vi "Resize Image for Question.vi"(8 "error in (no error)":errorcluster, 11 "Controller in":refnum<class "Controller.lvclass">) -> (0 "error out":errorcluster, 3 "Controller Out":refnum<class "Controller.lvclass">)   [LabVIEW 2024, in "Controller.lvlib" / "Controller.lvclass"]
uses:
  Controller.lvclass
  Controller.lvclass/Controller.ctl
  <vilib>/picture/picture.llb/Draw True-Color Pixmap.vi
  <vilib>/Dataflow_G/G-Image/Image Processing/Polymorphic VIs/Resize Image (Scale).vi
  <vilib>/Dataflow_G/G-Image/G-Image.lvlib
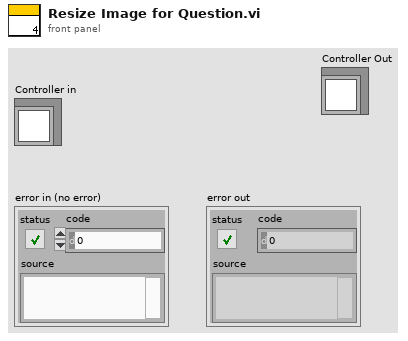
[diagram p1: front panel]
types:
  T1 = cluster{"horizontal":enum16{"left", "center", "right"}, "vertical":enum16{"top", "center", "bottom"}, "text":enum16{"left", "center", "right"}}
  T2 = enum16{"User-specified Font", "Application Font", "System Font", "Dialog Font"}
  T3 = cluster{"Font Name:":string, "Size":i16, "Strikeout?":bool, "Italic?":bool, "Underline?":bool, "Outline?":bool, "Shadow?":bool, "Bold?":bool}
  T4 = cluster{"left":i16, "top":i16, "right":i16, "bottom":i16}
  T5 = typedef "imagedata.ctl" = cluster{"image type":i32, "image depth":i32, "image":u8[], "mask":u8[], "colors":u32[], "Rectangle":cluster{"left":i16, "top":i16, "right":i16, "bottom":i16}}
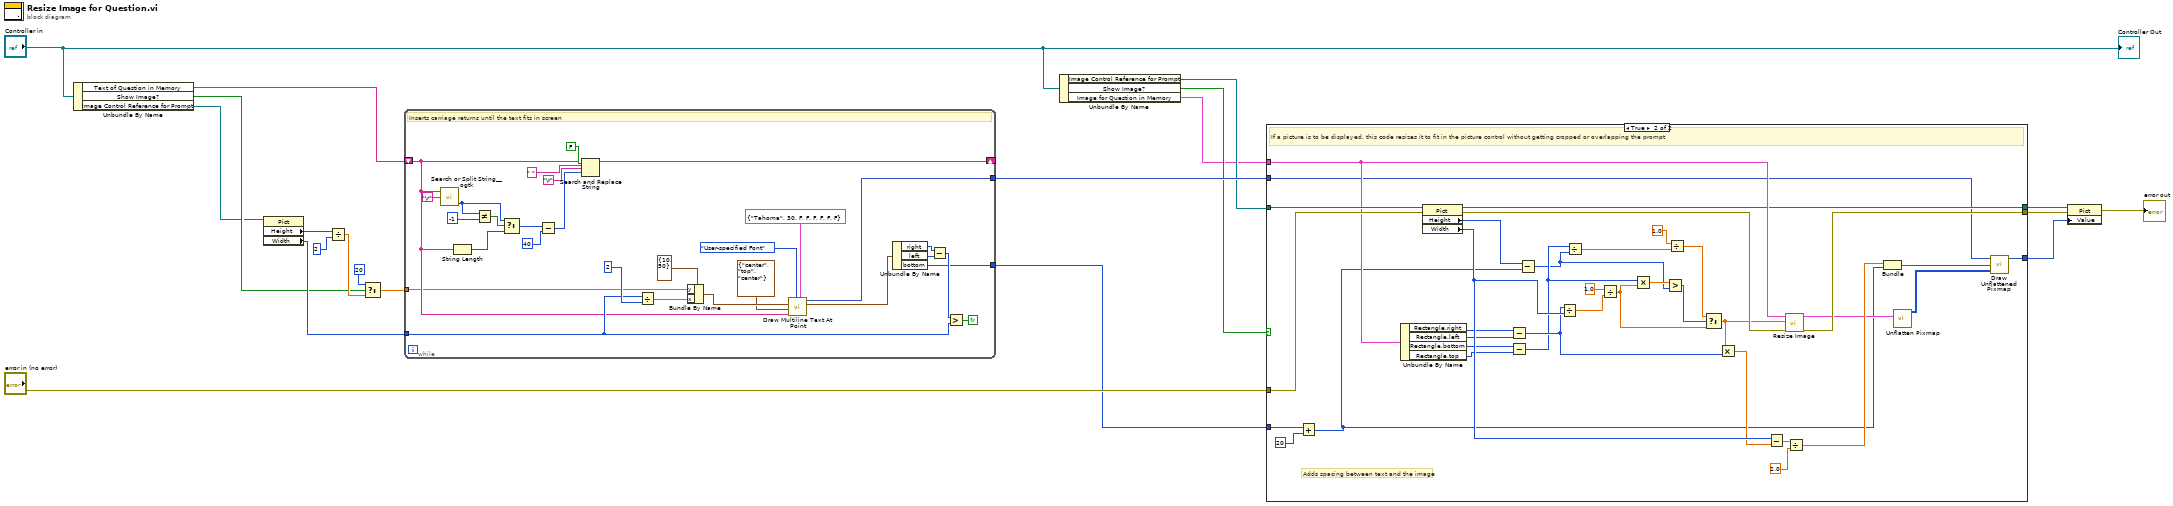
[diagram p0: block diagram]
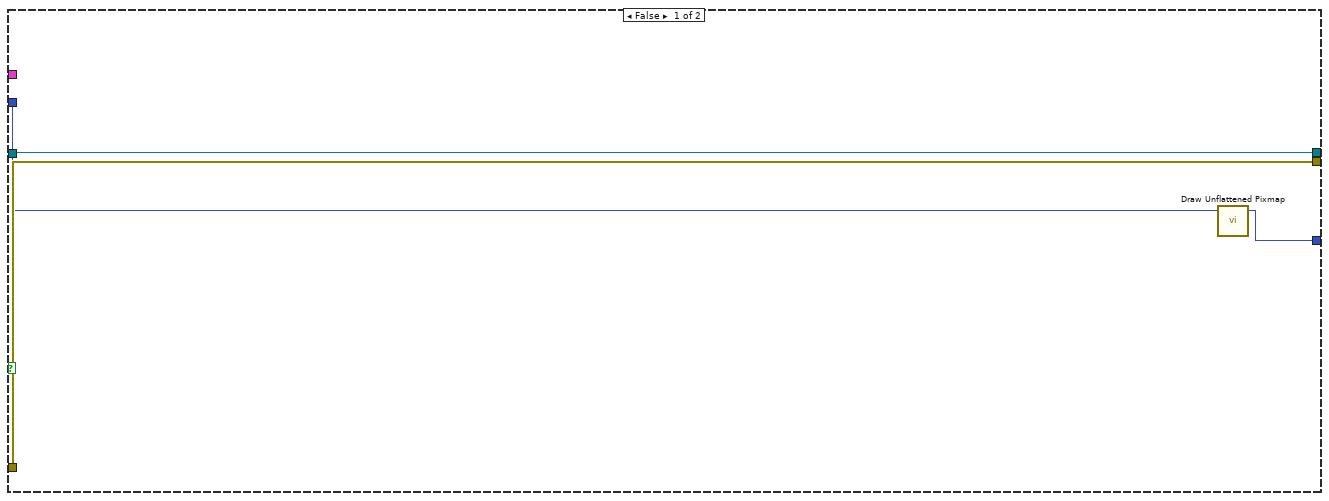
[diagram p2: hidden frame]
diagram:
  n1 = Unbundle By Name("Controller in") -> ("Text of Question in Memory"=w5:string, "Show Image?"=w4:bool, "Image Control Reference for Prompt"=w2:refnum<vi>)
  n2 = property class="Pict"(reference=w2) -> ("Height"=w8:u32, "Width"=w6:u32)  [unwired: 1 in, 2 out]
  n3 = Divide(x=w8, y=u32 2) -> (x/y=w7:dbl)
  n4 = Select(t=i16 20 ("x"), s=w4, f=w7) -> (s? t:f=w13:dbl)
  n5 = while {
    tunnel: [w49] -> w15
    tunnel: w6 -> [w39]
    shift-right: [w33] -> _
    shift-left: w5 -> [w31]
    tunnel: w13 -> [w21]
    tunnel: [w22] -> w11
    stop <- w42 continue-if-true
    # "Inserts carriage returns until the text fits in screen"
    n6 = call <userlib>:"Search or Split String__ogtk.vi"("search string/char (-)"="\r", "string"=w31) -> ("offset after match"=w25:i32)  [unwired: 1 in, 2 out]
    n7 = String Length(string=w31) -> (length=w26:i32)
    n8 = Not Equal?(x=w25, y=-1) -> (x != y?=w28:bool)
    n9 = Select(t=w25, s=w28, f=w26) -> (s? t:f=w24:i32)
    n10 = Subtract(x=w24, y=40 ("offset (0)")) -> (x-y=w27:i32)
    n11 = Search and Replace String(replace all?=FALSE ("replace all? (F)"), input string=w31, search string=" ", replace string="\r", offset=w27) -> (result string=w33:string)  [unwired: 3 in, 3 out]
    n12 = Divide(x=w39, y=u32 2) -> (x/y=w41:dbl)
    n13 = Bundle By Name(cluster=cluster{"x":i16, "y":i16} {"x"=10, "y"=50} ("origin"), "y"=w21, "x"=w41) -> (w37:cluster{"x":i16, "y":i16})
    n14 = call "Draw Multiline Text At Point.vi"("[user-specified font]"=T3 {"Font Name:"="Tahoma", "Size"=30, "Strikeout?"=FALSE, "Italic?"=FALSE, "Underline?"=FALSE, "Outline?"=FALSE, "Shadow?"=FALSE, "Bold?"=FALSE}, "desired font(Application)"=T2."User-specified Font", "text"=w31, "alignment(left, top,text)"=T1 {"horizontal"=enum."center", "vertical"=enum."top", "text"=enum."center"}, "origin"=w37) -> ("text rect"=w46:T4, "new picture"=w49:picture)  [unwired: 5 in]
    n15 = Unbundle By Name(w46) -> ("right"=w45:i16, "left"=w44:i16, "bottom"=w22:i16)
    n16 = Subtract(x=w45, y=w44) -> (x-y=w43:i16)
    n17 = Greater?(x=w43, y=w39) -> (0:w42:bool)
  }
  n18 = Unbundle By Name("Controller in") -> ("Image Control Reference for Prompt"=w14:refnum<vi>, "Show Image?"=w12:bool, "Image for Question in Memory"=w1:T5)
  n19 = case shown="True" w12 {
    tunnel: "error in (no error)" -> [w53 w89]
    tunnel: [w53 w88] -> w18
    tunnel: w14 -> [w52 w86]
    tunnel: w1 -> [_ w85]
    tunnel: [w52 w84] -> w17
    tunnel: w15 -> [w51 w62]
    tunnel: [w50 w59] -> w16
    tunnel: w11 -> [_ w56]
    frame False {
      n20 = call-poly <vilib>:"Draw Unflattened Pixmap.vi"("picture"=w51) -> ("new picture"=w50:picture)  [unwired: 8 in]
    }
    frame True {
      # "Adds spacing between text and the image"
      # "If a picture is to be displayed, this code resizes it to fit in the picture control without getting cropped or overlapping the prompt"
      n21 = Add(x=w56, y=i16 20) -> (x+y=w54:i16)
      n22 = Unbundle By Name(w85) -> ("Rectangle.right"=w63:i16, "Rectangle.left"=w64:i16, "Rectangle.bottom"=w75:i16, "Rectangle.top"=w76:i16)
      n23 = property class="Pict"(reference=w86, error in=w89) -> (reference out=w84:refnum<vi>, error out=w87:errorcluster, "Height"=w58:u32, "Width"=w80:u32)
      n24 = Subtract(x=w63, y=w64) -> (x-y=w77:i16)
      n25 = Subtract(x=w75, y=w76) -> (x-y=w74:i16)
      n26 = Subtract(x=w58, y=w54) -> (x-y=w57:u32)
      n27 = Divide(x=w77, y=w80) -> (x/y=w65:dbl)
      n28 = Divide(x=w74, y=w57) -> (x/y=w71:dbl)
      n29 = Divide(x=1.0, y=w65) -> (x/y=w69:dbl)
      n30 = Multiply(x=w74, y=w69) -> (x*y=w67:dbl)
      n31 = Greater?(x=w67, y=w57) -> (0:w68:bool)
      n32 = Divide(x=1.0, y=w71) -> (x/y=w73:dbl)
      n33 = Select(t=w73, s=w68, f=w69) -> (s? t:f=w78:dbl)
      n34 = Multiply(x=w78, y=w77) -> (x*y=w79:dbl)
      n35 = Subtract(x=w80, y=w79) -> (x-y=w81:dbl)
      n36 = call-poly <vilib>:"Resize Image.vi"("error in (no error)"=w87, "Scale"=w78, "Image"=w85) -> ("error out"=w88:errorcluster, "Resized Image"=w72:T5)  [unwired: 7 in]
      n37 = Divide(x=w81, y=2.0) -> (x/y=w82:dbl)
      n38 = Bundle(w82, w54) -> (w61:cluster{dbl, i16})  [unwired: 1 in]
      n39 = call <vilib>:"Unflatten Pixmap.vi"("image data"=w72) -> ("24-bit pixmap"=w60:u32[][])  [unwired: 4 in, 6 out]
      n40 = call-poly <vilib>:"Draw Unflattened Pixmap.vi"("picture"=w62, "top left point(0, 0)"=w61, "data (RGB format)"=w60) -> ("new picture"=w59:picture)  [unwired: 6 in]
    }
  }
  n41 = property class="Pict"(reference=w17, error in=w18, "Value"=w16) -> (error out=→"error out":errorcluster)  [unwired: 1 out]
  "Controller Out" <- "Controller in"
